vi "SetDisplayDataChartDialogTitle.vi"(8 "Error In":errorcluster, 10 "Chart Settings":T1={"Live SMU"=enum."A", "Live DUT"=1, "Live Measure Value"=enum."Voltage"} {"Live DUT" min=1 step=1}, 11 "VI Ref In":refnum<vi>) -> (0 "Error Out":errorcluster, 3 "VI Ref Out":refnum<vi>)   [LabVIEW 2012]
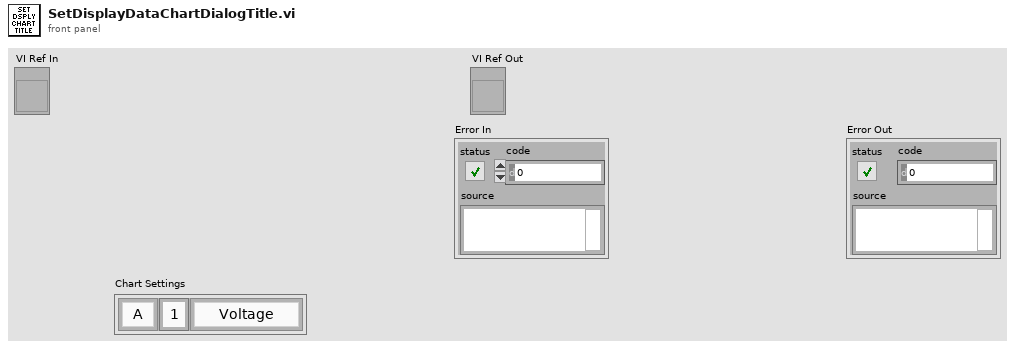
[diagram p1: front panel]
types:
  T1 = cluster{"Live SMU":enum16{"A", "B"}, "Live DUT":u32, "Live Measure Value":enum16{"Voltage", "Current", "Resistance"}}
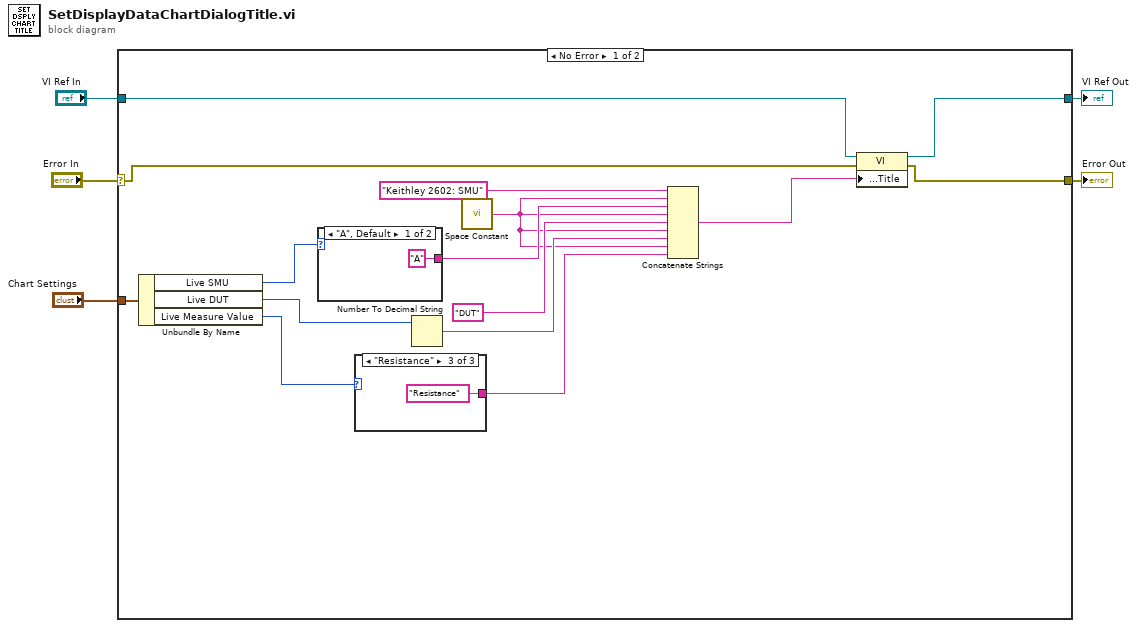
[diagram p0: block diagram]
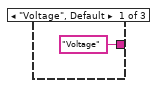
[diagram p2: hidden frame]
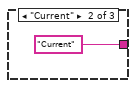
[diagram p3: hidden frame]
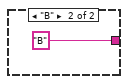
[diagram p4: hidden frame]
diagram:
  n1 = case shown="No Error" "Error In" {
    selector: "Error In" -> [w9 w27]
    tunnel: [w8 w27] -> w4
    tunnel: "Chart Settings" -> [w13 _]
    tunnel: "VI Ref In" -> [w7 w26]
    tunnel: [w6 w26] -> w1
    frame No Error {
      n2 = Unbundle By Name(w13) -> ("Live SMU"=w12:enum16{"A", "B"}, "Live DUT"=w11:u32, "Live Measure Value"=w10:enum16{"Voltage", "Current", "Resistance"})
      n3 = case shown="\"A\", Default" w12 {
        tunnel: ["A" "B"] -> w19
        frame "A", Default {
        }
        frame "B" {
        }
      }
      n4 = case shown="\"Resistance\"" w10 {
        tunnel: ["Voltage" "Current" "Resistance"] -> w15
        frame "Voltage", Default {
        }
        frame "Current" {
        }
        frame "Resistance" {
        }
      }
      n5 = Number To Decimal String(number=w11) -> (decimal integer string=w17:string)  [unwired: 1 in]
      n6 = call <vilib>:"Space Constant.vi"() -> ("String"=w16:string)
      n7 = Concatenate Strings("Keithley 2602: SMU", w16, w19, w16, "DUT", w16, w17, w16, w15) -> (w14:string)
      n8 = property class="VI"(reference=w7, error in=w9, "Front Panel.Title"=w14) -> (reference out=w6:refnum<vi>, error out=w8:errorcluster)
    }
    frame Error {
    }
  }
  "Error Out" <- w4
  "VI Ref Out" <- w1
